vi "File Path Creation.vi"(8 "ErrorIN":errorcluster, 9 "DL PrivateDataIN":refnum<class "DataLogger.lvclass">, 10 "State":string, 11 "LocalDataIN":T1) -> (0 "ErrorOUT":errorcluster, 3 "LocalDataOUT":T1)   [LabVIEW 2019, in "DataLogger.lvclass"]
uses:
  DataLogger.lvclass
  Common/Controls/AllPartInfo.ctl
  <vilib>/vision/Image Controls.llb/IMAQ Image.ctl
  Controls/LocalData_DL.ctl
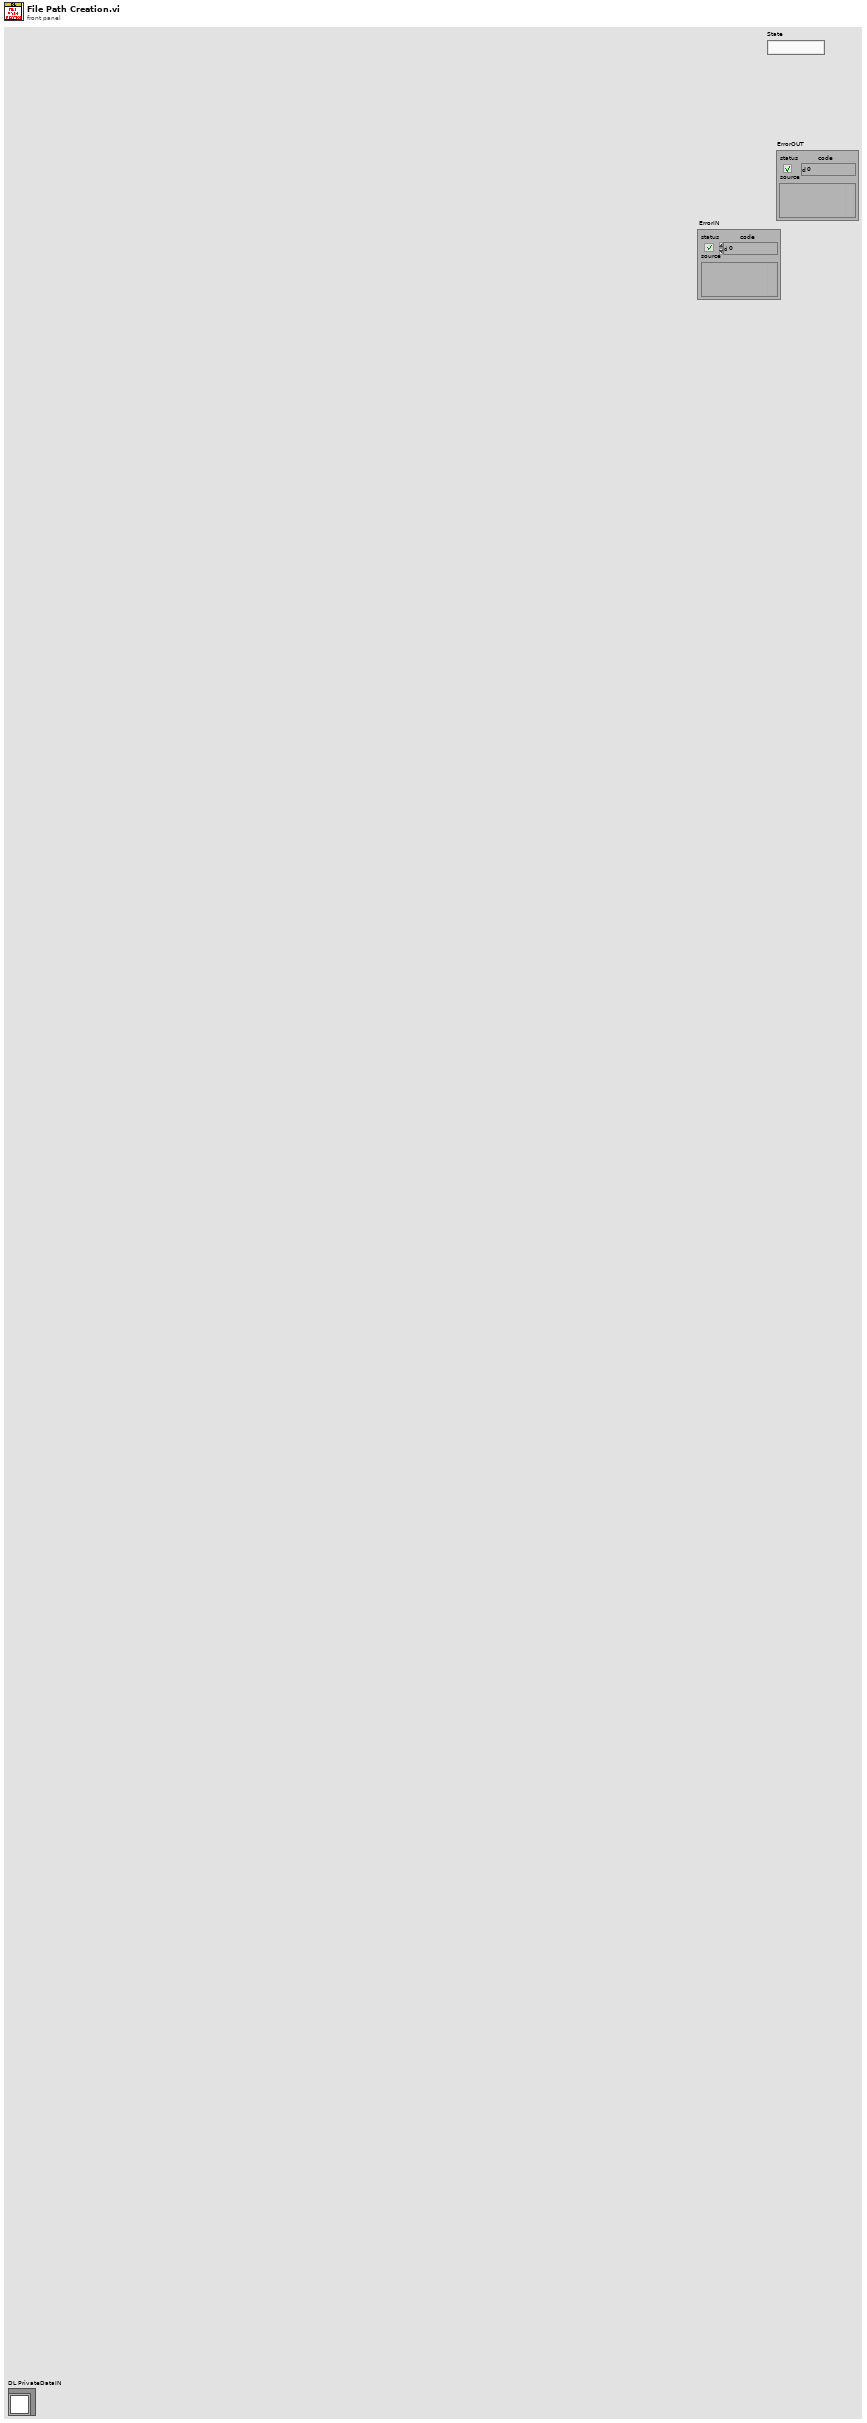
[diagram p1: front panel]
types:
  T1 = typedef "DataLogger.lvclass/LocalData_DL.ctl" = cluster{"Core":cluster{"Current VI Reference":refnum<vi>, "Close Panel on Exit?":bool}, "System Info":cluster{"System Name":string, "System ID":string, "Version":string, "Year":string, "Customer Details":cluster{"Customer Name":string, "Customer ID":string, "Location":string, "No of Shifts":u8, "Shift Details Array":cluster{"Name":string, "Timing":string}[]}, "Software Features":cluster{"IoT Enable":bool, "Datalogging Features":cluster{"Event Data":bool, "Measurement Data":bool, "Statistical Data":bool, "Reel Data":bool, "Failed Measurement Data":bool, "Failed Images":bool}, "IoT":cluster{"SMS Alert Enable":bool, "Email Alert Enable":bool}, "Popup Enable?":cluster{"Fail":bool, "Pause":bool, "Stop":bool}}}, "Part Info":cluster{"Part Name":string, "Rack ID":u8, "Initialize":bool, "StampingMc No":u64, "Operator Name":string, "ReelCount":u64, "TotalCount":u64, "Measurement Names Array":string[], "Measurement ID Array":u16[], "Spec Values Array":cluster{"LCL":dbl, "UCL":dbl, "LSL":dbl, "USL":dbl, "Nominal Value":dbl}[], "Camera Name Array":string[], "Measurement Enable/Disable Array":bool[], "Number of Measurements":i32}, "Fail Counter(For Event Details)":i32, "Event Details":cluster{"Event Name":string, "Event Time":string, "Event Reason":string, "Previous Event Name":string, "Previous Event Time":string}, "StatisticalInfo":string[][], "BatchInfo":cluster{"BatchPassCount":u64, "BatchFailCount":u64}, "Failure Details":cluster{"Fail Time Stamp":u64, "ControlPFArray":bool[], "SpecificationPFArray":dbl[], "Rack ID":u8, "Failed Image Array":T2[], "Fail Date":string, "Fail Time":string, "Fail Reason":string}, "SaveFailedImageCounter":i32, "AllPartInfoArray":T3, "Status":bool, "SpecValues(ForUpdate)":cluster{"LCL":dbl, "UCL":dbl, "LSL":dbl, "USL":dbl, "Nominal Value":dbl}, "AddSuccessfull":bool, "CurrentStateMessage":string, "IoTDetailsCounter":bool, "InitialUpdate":bool, "ResetUpdate":bool, "SetCounter":cluster{"MeasurementDetailsSetCounter":i32, "BatchDetailsSetCounter":i32, "FailureDetailsSetCounter":i32, "EventDetailsSetCounter":i32}, "IndexCounter":cluster{"MeasurementDetailsIndexCounter":i32, "BatchDetailsIndexCounter":i32, "FailureDetailsIndexCounter":i32, "EventDetailsIndexCounter":i32}, "Details2D":cluster{"MeasurementDetails(2D)":string[][], "BatchDetails(2D)":string[][], "FailureDetails(2D)":string[][], "EventDetails(2D)":string[][]}, "IDs":cluster{"Stamping McID":string, "Inspection McID":string, "BatchID":string, "FailID":string}, "Reel Info":cluster{"Reel No":u64, "Reel Start Time Stamp":u64}, "ExcelData":cluster{"StripPath":bool, "ReelCounterPerPart":i32, "FilePaths":cluster{"EventsFilePath":path, "FailFilePath":path, "ReelFilePath":path, "StatisticalFilePath":path}, "ExcelSheetCounterPerReel":cluster{"EventsSheetCounter":u32, "FailSheetCounter":u32, "StatisticalSheetCounter":u32, "ReelSheetCounter":u32}, "CreateNewExcel":cluster{"CreateNewEventsExcel":bool, "CreateNewFailExcel":bool, "CreateNewStatisticalExcel":bool, "CreateNewReelExcel":bool}, "RecordsInExcelCounter":cluster{"EventsRecordsCounter":u32, "FailRecordsCounter":u32, "ReelRecordsCounter":u32, "StatisticalRecordsCounter":u32}}, "SaveAck":cluster{"Loop1":bool, "Loop2":bool}, "Shift Statistical Info":cluster{"Shift Name":string, "Shift Timing":string, "Shift End Date":string, "Statistical Shift Data":cluster{"PartName":string, "MeasurementNames":string[], "Statistical Parameters":string[][]}[]}}
  T2 = typedef "IMAQ Image.ctl" = refnum<image>
  T3 = typedef "AllPartInfo.ctl" = cluster{"PartName":string, "NumberOfRacks":u8, "MeasurementIDsArray":u16[], "MeasurementNamesArray":string[], "SpecValuesArray":cluster{"LCL":dbl, "UCL":dbl, "LSL":dbl, "USL":dbl, "NominalValue":dbl}[]}[]
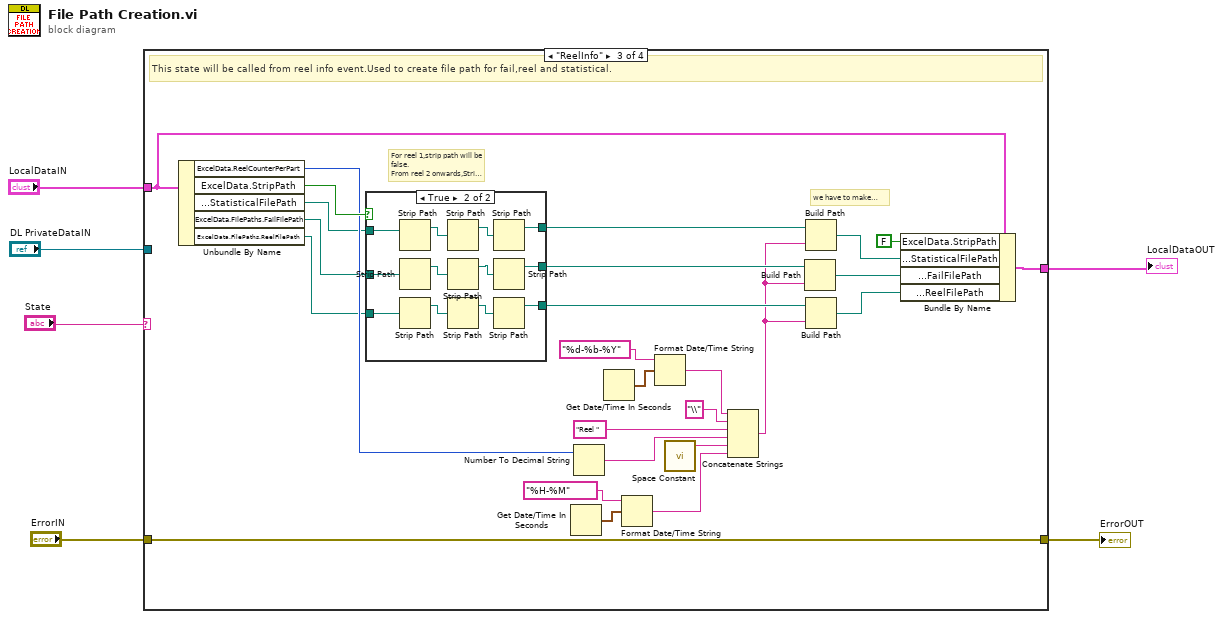
[diagram p0: block diagram]
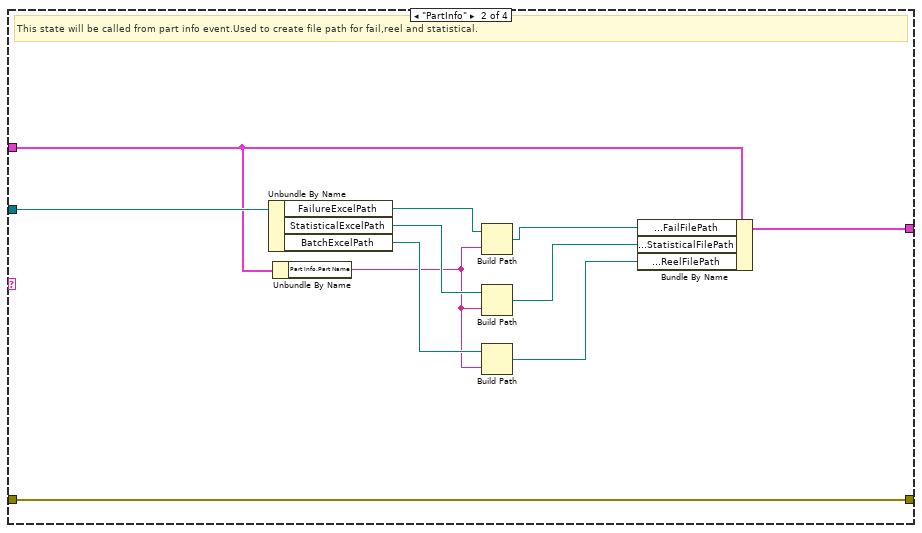
[diagram p3: hidden frame]
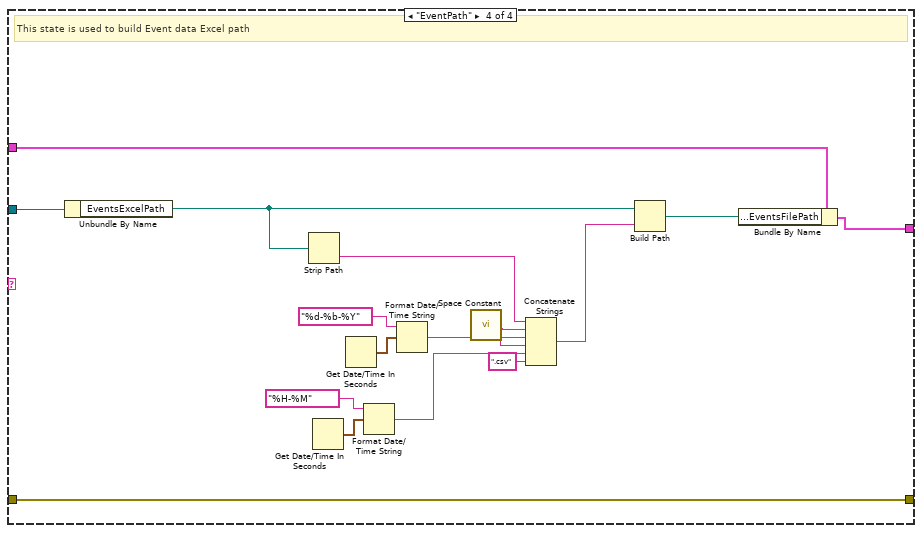
[diagram p5: hidden frame]
diagram:
  n1 = case shown="\"ReelInfo\"" "State" {
    tunnel: "LocalDataIN" -> [w8 w18 w26 w65]
    tunnel: "DL PrivateDataIN" -> [_ w19 _ w71]
    tunnel: [w8 w17 w22 w63] -> w4
    tunnel: [w7 w9 w21 w62] -> w2
    tunnel: "ErrorIN" -> [w7 w9 w21 w62]
    frame Default {
    }
    frame "PartInfo" {
      # "This state will be called from part info event.Used to create file path for fail,reel and statistical."
      n2 = Unbundle By Name(w19) -> ("FailureExcelPath"=w16:path, "StatisticalExcelPath"=w15:path, "BatchExcelPath"=w14:path)
      n3 = Unbundle By Name(w18) -> ("Part Info.Part Name"=w13:string)
      n4 = Build Path(base path=w16, name or relative path=w13) -> (appended path=w12:path)
      n5 = Build Path(base path=w15, name or relative path=w13) -> (appended path=w11:path)
      n6 = Build Path(base path=w14, name or relative path=w13) -> (appended path=w10:path)
      n7 = Bundle By Name(cluster=w18, "ExcelData.FilePaths.FailFilePath"=w12, "ExcelData.FilePaths.StatisticalFilePath"=w11, "ExcelData.FilePaths.ReelFilePath"=w10) -> (w17:T1)
    }
    frame "ReelInfo" {
      # "we have to make strip path false otherwise path will again be stripped(which we dont want) \nin ExcelFoldercreation SubVI."
      # "For reel 1,strip path will be false.\nFrom reel 2 onwards,Strip path was true.So some path is stripped."
      # "This state will be called from reel info event.Used to create file path for fail,reel and statistical."
      n8 = Unbundle By Name(w26) -> ("ExcelData.ReelCounterPerPart"=w33:i32, "ExcelData.StripPath"=w34:bool, "ExcelData.FilePaths.StatisticalFilePath"=w32:path, "ExcelData.FilePaths.FailFilePath"=w31:path, "ExcelData.FilePaths.ReelFilePath"=w30:path)
      n9 = case shown="True" w34 {
        tunnel: w32 -> [w48 w60]
        tunnel: [w48 w58] -> w39
        tunnel: w31 -> [w47 w55]
        tunnel: w30 -> [w46 w54]
        tunnel: [w47 w53] -> w29
        tunnel: [w46 w52] -> w28
        frame False {
        }
        frame True {
          n10 = Strip Path(path=w60) -> (stripped path=w59:path)  [unwired: 1 out]
          n11 = Strip Path(path=w55) -> (stripped path=w56:path)  [unwired: 1 out]
          n12 = Strip Path(path=w54) -> (stripped path=w51:path)  [unwired: 1 out]
          n13 = Strip Path(path=w59) -> (stripped path=w57:path)  [unwired: 1 out]
          n14 = Strip Path(path=w56) -> (stripped path=w49:path)  [unwired: 1 out]
          n15 = Strip Path(path=w51) -> (stripped path=w50:path)  [unwired: 1 out]
          n16 = Strip Path(path=w57) -> (stripped path=w58:path)  [unwired: 1 out]
          n17 = Strip Path(path=w49) -> (stripped path=w53:path)  [unwired: 1 out]
          n18 = Strip Path(path=w50) -> (stripped path=w52:path)  [unwired: 1 out]
        }
      }
      n19 = Get Date/Time In Seconds() -> (seconds since 1Jan1904=w43:timestamp)
      n20 = Number To Decimal String(number=w33) -> (decimal integer string=w44:string)  [unwired: 1 in]
      n21 = Get Date/Time In Seconds() -> (seconds since 1Jan1904=w38:timestamp)
      n22 = Format Date/Time String(time format string (%c)="%H-%M", seconds (now)=w43) -> (date/time string=w40:string)  [unwired: 1 in]
      n23 = Format Date/Time String(time format string (%c)="%d-%b-%Y", seconds (now)=w38) -> (date/time string=w36:string)  [unwired: 1 in]
      n24 = call <vilib>:"Space Constant.vi"() -> ("String"=w41:string)
      n25 = Concatenate Strings(w36, "\\" ("string"), "Reel ", w44, w41, w40) -> (w27:string)
      n26 = Build Path(base path=w29, name or relative path=w27) -> (appended path=w24:path)
      n27 = Build Path(base path=w39, name or relative path=w27) -> (appended path=w25:path)
      n28 = Build Path(base path=w28, name or relative path=w27) -> (appended path=w23:path)
      n29 = Bundle By Name(cluster=w26, "ExcelData.StripPath"=FALSE, "ExcelData.FilePaths.StatisticalFilePath"=w25, "ExcelData.FilePaths.FailFilePath"=w24, "ExcelData.FilePaths.ReelFilePath"=w23) -> (w22:T1)
    }
    frame "EventPath" {
      # "This state is used to build Event data Excel path"
      n30 = Unbundle By Name(w71) -> ("EventsExcelPath"=w61:path)
      n31 = Strip Path(path=w61) -> (name=w70:string)  [unwired: 1 out]
      n32 = Get Date/Time In Seconds() -> (seconds since 1Jan1904=w73:timestamp)
      n33 = Get Date/Time In Seconds() -> (seconds since 1Jan1904=w76:timestamp)
      n34 = Format Date/Time String(time format string (%c)="%H-%M", seconds (now)=w73) -> (date/time string=w68:string)  [unwired: 1 in]
      n35 = Format Date/Time String(time format string (%c)="%d-%b-%Y", seconds (now)=w76) -> (date/time string=w72:string)  [unwired: 1 in]
      n36 = call <vilib>:"Space Constant.vi"() -> ("String"=w69:string)
      n37 = Concatenate Strings(w70, w69, w72, w69, w68, ".csv" ("string")) -> (w66:string)
      n38 = Build Path(base path=w61, name or relative path=w66) -> (appended path=w64:path)
      n39 = Bundle By Name(cluster=w65, "ExcelData.FilePaths.EventsFilePath"=w64) -> (w63:T1)
    }
  }
  "LocalDataOUT" <- w4
  "ErrorOUT" <- w2
